vi "MTM2_getEvent_cellTemperatureHiWarning.vi"(8 "error in (no error)":errorcluster, 11 "logevent_cellTemperatureHiWarning_Ctl":T1) -> (0 "error out":errorcluster, 2 "function return":i32, 3 "logevent_cellTemperatureHiWarning_Ctl out":T1)   [LabVIEW 2018, in "SALLV_MTM2.lvlib"]
doc: "int MTM2_shm_getEvent_cellTemperatureHiWarningLV(MTM2_logevent_cellTemperatureHiWarningLV *logevent_cellTemperatureHiWarning_Ctl );"
uses:
  DataTypes/logevent_cellTemperatureHiWarning.ctl
  SALLV_MTM2.lvlib
  SALLV_MTM2.so
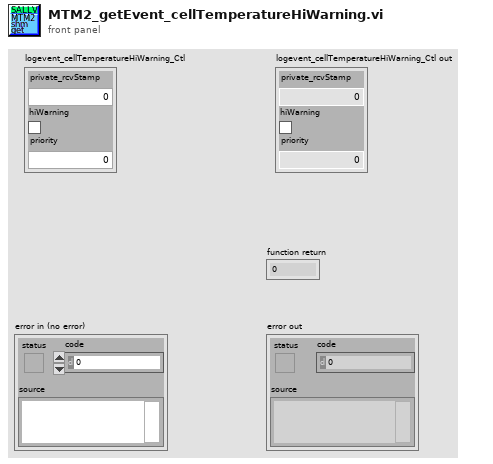
[diagram p1: front panel]
types:
  T1 = typedef "SALLV_MTM2.lvlib/logevent_cellTemperatureHiWarning.ctl" = cluster{"private_rcvStamp":dbl, "hiWarning":bool, "priority":i32}
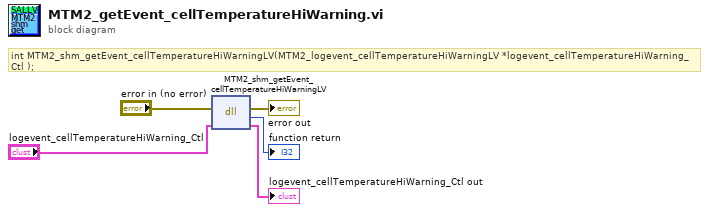
[diagram p0: block diagram]
diagram:
  # "int MTM2_shm_getEvent_cellTemperatureHiWarningLV(MTM2_logevent_cellTemperatureHiWarningLV *logevent_cellTemperatureHiWarning_Ctl );"
  n1 = dll-call lib="home/ttsai/Documents/salLabviewApi/SALLV_MTM2/SALLV_MTM2.*" fn="MTM2_shm_getEvent_cellTemperatureHiWarningLV"(error in="error in (no error)", "logevent_cellTemperatureHiWarning_Ctl"="logevent_cellTemperatureHiWarning_Ctl") -> (error out=→"error out":errorcluster, →"function return":i32, "logevent_cellTemperatureHiWarning_Ctl"=→"logevent_cellTemperatureHiWarning_Ctl out":T1)  [unwired: 2 in, 1 out]
